vi "poly_control_value_from_name_multi.vi"(8 "error in (no error)":errorcluster, 10 "control names":string[](array[string]), 11 "vi ref":refnum<vi>) -> (0 "error out":errorcluster, 1 "Types":T1[](array[typedef]), 2 "Values":variant[](array[variant]), 3 "vi ref dup":refnum<vi>, 4 "found?":bool[](array[boolean]), 5 "ctrl refs":refnum<vi>[](array[refnum]))   [LabVIEW 2015, in "_ref_tools_polys.lvlib"]
uses:
  _ref_tools_polys.lvlib
  <vilib>/Utility/Data Type/Type Definitions/Data Type.ctl
  poly_control_ref_from_name_multi.vi
  <vilib>/Utility/Data Type/NI_Data Type.lvlib
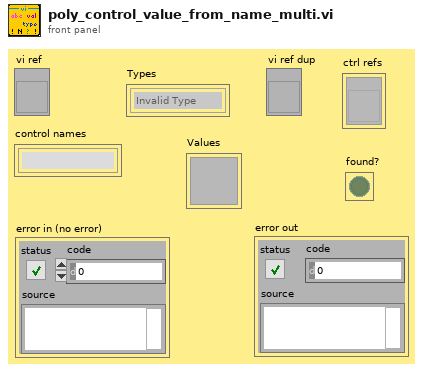
[diagram p1: front panel]
types:
  T1 = typedef "NI_Data Type.lvlib/Data Type.ctl" = enum8{"Invalid Type", "Void", "I8", "I16", "I32", "I64", "U8", "U16", "U32", "U64", "Single Float", "Double Float", "Extended Float", "Single Complex", "Double Complex", "Extended Complex", "Enum U8", "Enum U16", "Enum U32", "Enum U64", "Single Float With Unit", "Double Float With Unit", "Extended Float With Unit", "Single Complex with Unit", "Double Complex with Unit", "Extended Complex with Unit", "Boolean", "String", "Path", "Picture", "Tag", "Array", "Cluster", "Variant", "LV Variant", "Waveform", "Timestamp", "Digital Waveform", "Digital Data", "ExpressData", "Refnum", "External Data", "VI", "Poly VI", "LabVIEW Class Instance", "Fixed Point"}
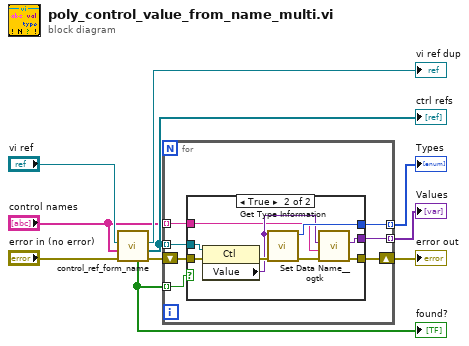
[diagram p0: block diagram]
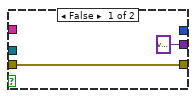
[diagram p2: hidden frame]
diagram:
  n1 = call-poly "control_ref_form_name.vi"("error in (no error)"="error in (no error)", "control names"="control names", "vi ref"="vi ref") -> ("error out"=w7:errorcluster, "ctrl refs"=w2:refnum<vi>[], "vi ref dup"=→"vi ref dup":refnum<vi>, "found?"=w4:bool[])  [unwired: 5 in]
  "ctrl refs" <- w2
  "found?" <- w4
  n2 = for {
    shift-right: [w16] -> w6
    shift-left: w7 -> [w17]
    tunnel: [w15] -> w5 mode=indexing
    tunnel: w4 -> [w14] mode=indexing
    tunnel: [w13] -> w3 mode=indexing
    tunnel: w2 -> [w12] mode=indexing
    tunnel: "control names" -> [w11] mode=indexing
    n3 = case shown="True" w14 {
      tunnel: w17 -> [w18 w28]
      tunnel: [w18 w20] -> w16
      tunnel: [variant w23] -> w15
      tunnel: [_ w26] -> w13
      tunnel: w12 -> [_ w25]
      tunnel: w11 -> [_ w22]
      frame False {
      }
      frame True {
        n4 = property class="Ctl"(reference=w25, error in=w28) -> (error out=w27:errorcluster, "Value"=w24:variant)  [unwired: 1 out]
        n5 = call <vilib>:"Get Type Information.vi"("error in (no error)"=w27, "Variant"=w24) -> ("error out"=w21:errorcluster, "Type"=w26:T1)  [unwired: 5 in, 3 out]
        n6 = call <userlib>:"Set Data Name__ogtk.vi"("error in (no error)"=w21, "Data Name"=w22, "Data"=w24) -> ("error out"=w20:errorcluster, "Renamed Data"=w23:variant)  [unwired: 7 in]
      }
    }
  }
  "error out" <- w6
  "Types" <- w3
  "Values" <- w5
